vi "Run_Post Core.vi"(0 "For Loop in":refnum<class "Structure Loop.lvclass">, 11 "error in (no error)":errorcluster) -> (4 "For Loop out":refnum<class "Structure Loop.lvclass">, 6 "Go to Run Pre Core?":bool, 15 "error out":errorcluster)   [LabVIEW 2019, in "Structure Loop.lvclass"]
uses:
  Structure Loop.lvclass
  Structure Loop.lvclass/Structure Loop.ctl
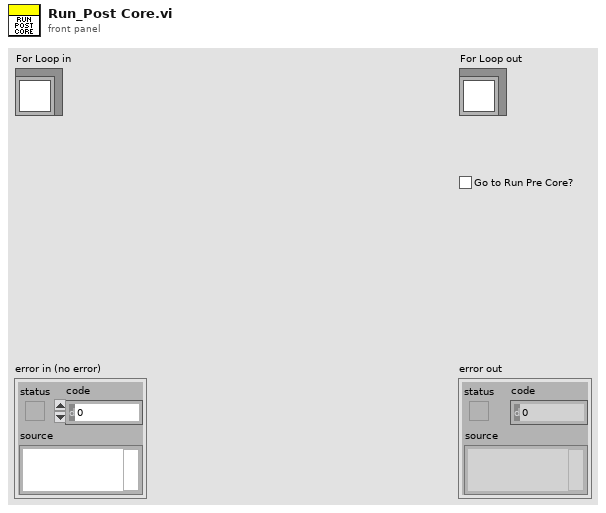
[diagram p1: front panel]
types:
  T1 = typedef "Structure Loop.lvclass/Function List.ctl" = enum16{"For Loop", "While Loop"}
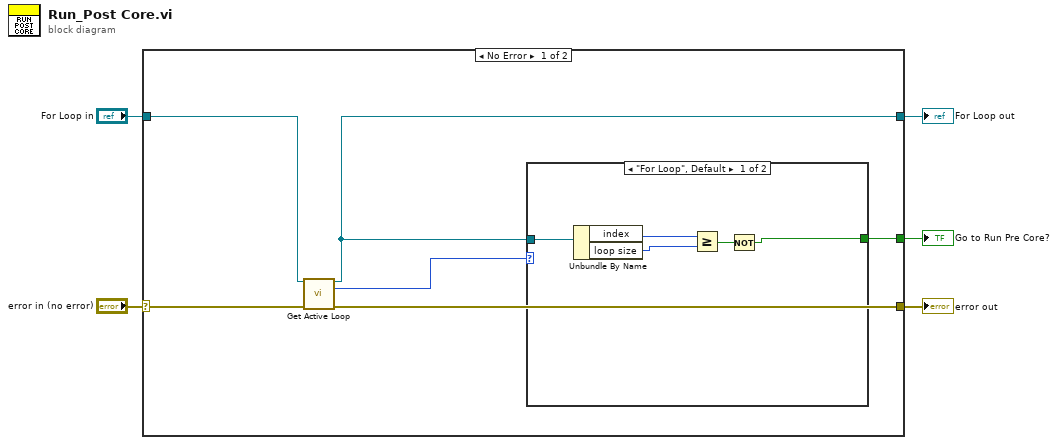
[diagram p0: block diagram]
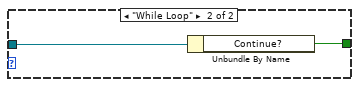
[diagram p2: hidden frame]
diagram:
  n1 = case shown="No Error" "error in (no error)" {
    selector: "error in (no error)" -> [w8 w20]
    tunnel: "For Loop in" -> [w7 w19]
    tunnel: [w10 w20] -> w4
    tunnel: [w9 w19] -> w2
    tunnel: [w11 _] -> w1
    frame No Error {
      n2 = call "Get Active Loop.vi"("Structure Loop in"=w7, "error in (no error)"=w8) -> ("Structure Loop out"=w9:refnum<class "Structure Loop.lvclass">, "Function List"=w6:T1, "error out"=w10:errorcluster)  [unwired: 11 in]
      n3 = case shown="\"For Loop\", Default" w6 {
        tunnel: [w12 w18] -> w11
        tunnel: w9 -> [w16 w17]
        frame "For Loop", Default {
          n4 = Unbundle By Name(w16) -> ("index"=w15:i32, "loop size"=w14:i32)
          n5 = Greater Or Equal?(x=w15, y=w14) -> (x >= y?=w13:bool)
          n6 = Not(x=w13) -> (.not. x?=w12:bool)
        }
        frame "While Loop" {
          n7 = Unbundle By Name(w17) -> ("Continue?"=w18:bool)
        }
      }
    }
    frame Error {
    }
  }
  "error out" <- w4
  "For Loop out" <- w2
  "Go to Run Pre Core?" <- w1
